vi "DangerZone(ElevatorWrist).vi"(2 "Wrist":T2(ring), 3 "Level":T1(ring)) -> (0 "Wrist":T2(ring), 1 "Level":T1(ring))   [LabVIEW 2018]
uses:
  <vilib>/Rock Robotics/WPI/ThirdParty/Phoenix-LabVIEW/Motor Controller/Get/CTRE_Phoenix_MotorController_GetSelectedSensorData.vi
panel:
  in  "Intake Lower Danger":i32
  in  "Intake Upper Danger":i32
  in  "Elevator Lower Danger":i32
  in  "Elevator Upper Danger":i32
  in  "Intake Lower Danger GO TO Cargoship":i32
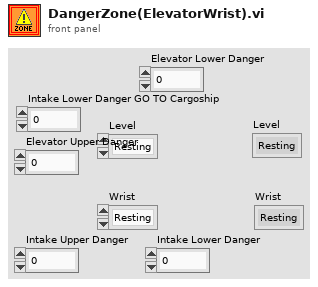
[diagram p1: front panel]
types:
  T1 = enum16{"Resting", "CargoShip Front", "CargoShip Back", "Cargo Mid", "Hatch Mid", "All High"}
  T2 = enum16{"Resting", "Hatch Ground Intake", "Hatch Place Low/Mid/CargoShip", "Hatch Place High", "Cargo Ground Intake", "Cargo Place Low/Mid", "Cargo Place High", "CargoShip Place Front", "CargoShip Place Back"}
  T3 = typedef "WPI_MotorControlDeviceRef.ctl" = cluster{"DeviceStatus":errorcluster, "Type":T4, "PWM":cluster{"PWM Channel":T5, "DeadBand":T6}, "CAN":cluster{"Device Number":u8, "SetOutput VI Ref":variant, "GetOutput VI Ref":variant, "Enable VI Ref":variant, "Disable VI Ref":variant, "Data":variant}, "Invert":bool, "DIO PWM":cluster{"PWM \"Enable\" Channel":T5, "DIOChannel":T7, "PWM Rate":dbl}}
  T4 = typedef "WPI_MotorControlType.ctl" = enum16{"PWM", "CAN", "DIO PWM"}
  T5 = typedef "FPGA_DIOPWMChannel.ctl" = enum8{"PWM 0", "PWM 1", "PWM 2", "PWM 3", "PWM 4", "PWM 5", "PWM 6", "PWM 7", "PWM 8", "PWM 9", "PWM MXP 0", "PWM MXP 1", "PWM MXP 2", "PWM MXP 3", "PWM MXP 4", "PWM MXP 5", "PWM MXP 6", "PWM MXP 7", "PWM MXP 8", "PWM MXP 9", "Invalid"}
  T6 = typedef "WPI_PWMDeadband.ctl" = cluster{"Name":string, "maxPositivePwm":i32, "minPositivePwm":i32, "centerPwm":i32, "maxNegativePwm":i32, "minNegativePwm":i32, "angularRange":u16}
  T7 = typedef "FPGA_DIOChannel.ctl" = enum8{"DIO 0", "DIO 1", "DIO 2", "DIO 3", "DIO 4", "DIO 5", "DIO 6", "DIO 7", "DIO 8", "DIO 9", "DIO MXP 0", "DIO MXP 1", "DIO MXP 2", "DIO MXP 3", "DIO MXP 4", "DIO MXP 5", "DIO MXP 6", "DIO MXP 7", "DIO MXP 8", "DIO MXP 9", "DIO MXP 10", "DIO MXP 11", "DIO MXP 12", "DIO MXP 13", "DIO MXP 14", "DIO MXP 15", "SPI Port CS1", "SPI Port CS2", "SPI Port CS3", "SPI Port MISO", "SPI Port MOSI", "Invalid"}
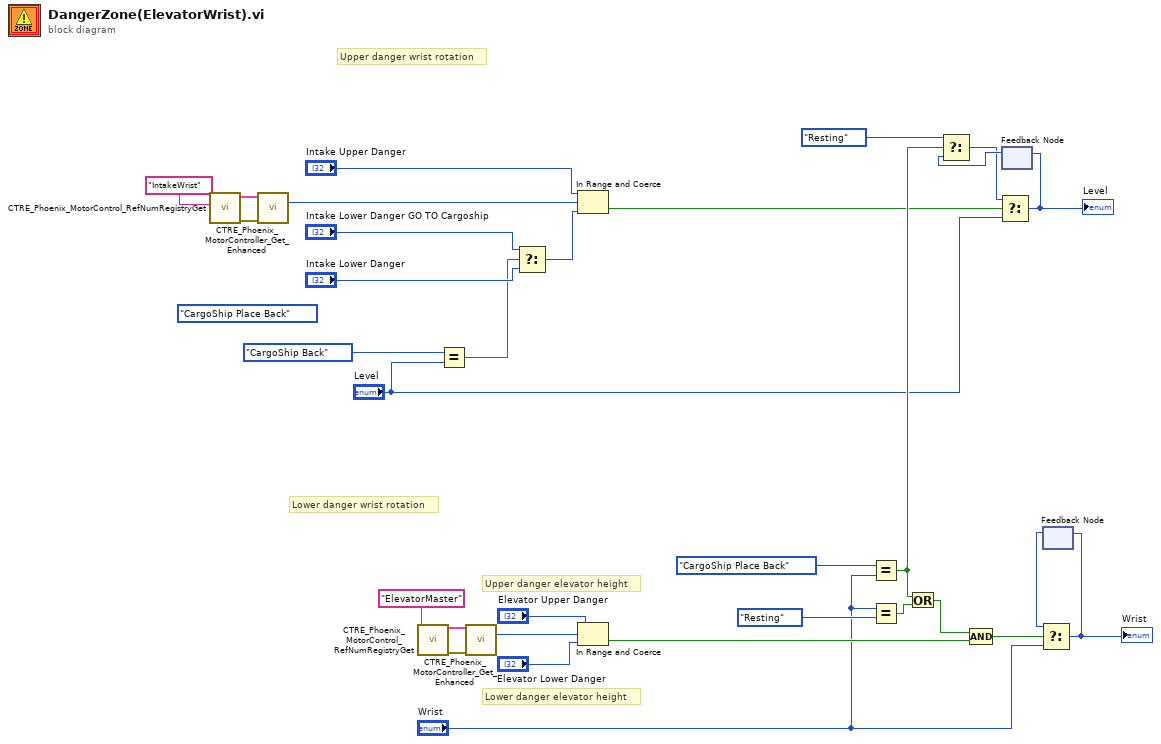
[diagram p0: block diagram]
diagram:
  (unwired) T2."CargoShip Place Back" ("Wrist 2")
  # "Lower danger elevator height"
  # "Upper danger wrist rotation"
  # "Lower danger wrist rotation"
  # "Upper danger elevator height"
  n1 = call <vilib>:"CTRE_Phoenix_MotorControl_RefNumRegistryGet.vi"("refnum name"="IntakeWrist") -> ("error out"=w31:errorcluster, "PhoenixMotorControlDevRef"=w30:T3)  [unwired: 9 in]
  n2 = call-poly <vilib>:"CTRE_Phoenix_MotorController_Get_Enhanced.vi"("PhoenixMotorControlDevRef"=w30, "error in"=w31) -> ("Position (Raw Sensor Units)"=w29:i32)  [unwired: 10 in, 3 out]
  n3 = call <vilib>:"CTRE_Phoenix_MotorControl_RefNumRegistryGet.vi"("refnum name"="ElevatorMaster") -> ("error out"=w27:errorcluster, "PhoenixMotorControlDevRef"=w26:T3)  [unwired: 9 in]
  n4 = Equal?(x=T1."CargoShip Back" ("f"), y="Level") -> (x = y?=w3:bool)
  n5 = call-poly <vilib>:"CTRE_Phoenix_MotorController_Get_Enhanced.vi"("PhoenixMotorControlDevRef"=w26, "error in"=w27) -> ("Position (Raw Sensor Units)"=w25:i32)  [unwired: 10 in, 3 out]
  n6 = Select(t="Intake Lower Danger GO TO Cargoship", s=w3, f="Intake Lower Danger") -> (s? t:f=w19:i32)
  n7 = In Range and Coerce(upper limit="Intake Upper Danger", x=w29, lower limit=w19) -> (In Range?=w4:bool)  [unwired: 1 out]
  n8 = In Range and Coerce(upper limit="Elevator Upper Danger", x=w25, lower limit="Elevator Lower Danger") -> (In Range?=w20:bool)  [unwired: 1 out]
  n9 = Equal?(x=T2."CargoShip Place Back" ("Wrist 2"), y="Wrist") -> (x = y?=w5:bool)
  n10 = Equal?(x="Wrist", y=T2."Resting" ("Wrist 2")) -> (x = y?=w10:bool)
  n11 = Or(x=w5, y=w10) -> (x .or. y?=w9:bool)
  n12 = Compound Arithmetic op=AND(w9, w20) -> (w15:bool)
  n13 = feedback #1() -> (w7:T1)  [unwired: 1 in]
  n14 = Select(t=T1."Resting" ("f"), s=w5, f=w7) -> (s? t:f=w6:T1)
  n15 = Select(t=w6, s=w4, f="Level") -> (s? t:f=w22:T1)
  "Level" <- w22
  n16 = feedback-in #1(w22) -> ()
  n17 = feedback #2() -> (w16:T2)  [unwired: 1 in]
  n18 = Select(t=w16, s=w15, f="Wrist") -> (s? t:f=w21:T2)
  "Wrist" <- w21
  n19 = feedback-in #2(w21) -> ()
